vi "Stop Sub-Panel VI.vi"(8 "error in (no error) 2":errorcluster, 11 "reference":refnum<vi>) -> (0 "error IO":errorcluster)   [LabVIEW 2011, in "PXIe-433x Custom Device.lvlib"]
uses:
  PXIe-433x Custom Device.lvlib
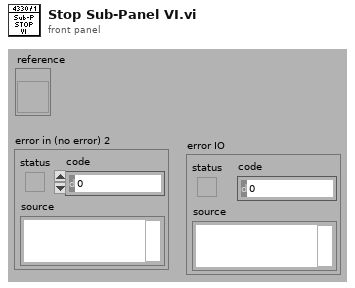
[diagram p1: front panel]
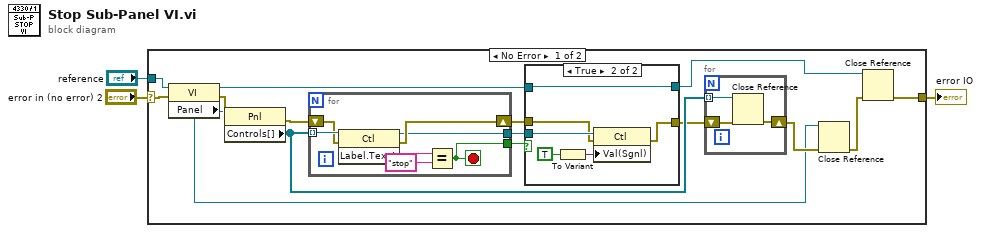
[diagram p0: block diagram]
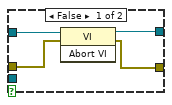
[diagram p2: hidden frame]
diagram:
  n1 = case shown="No Error" "error in (no error) 2" {
    selector: "error in (no error) 2" -> [w6 w39]
    tunnel: [w4 w39] -> w2
    tunnel: "reference" -> [w5 _]
    frame No Error {
      n2 = property class="VI"(reference=w5, error in=w6) -> (reference out=w13:refnum<vi>, error out=w18:errorcluster, "Panel"=w7:refnum<vi>)
      n3 = property class="Pnl"(reference=w7, error in=w18) -> (error out=w17:errorcluster, "Controls[]"=w12:refnum<vi>[])  [unwired: 1 out]
      n4 = for {
        tunnel: w12 -> [w38] mode=indexing
        tunnel: [w35] -> w14
        shift-right: [w33] -> w15
        shift-left: w17 -> [w34]
        tunnel: [w32] -> w16
        stop <- w35 stop-if-true
        n5 = property class="Ctl"(reference=w38, error in=w34) -> (reference out=w32:refnum<vi>, error out=w33:errorcluster, "Label.Text"=w37:string)
        n6 = Equal?(x=w37, y="stop") -> (x = y?=w35:bool)
      }
      n7 = case shown="True" w14 {
        tunnel: w16 -> [_ w31]
        tunnel: w15 -> [w24 w28]
        tunnel: w13 -> [w25 w26]
        tunnel: [w23 w26] -> w11
        tunnel: [w22 w27] -> w10
        frame False {
          n8 = invoke class="VI" method="Abort VI"(reference=w25, error in=w24) -> (reference out=w23:refnum<vi>, error out=w22:errorcluster)  [unwired: 1 in, 1 out]
        }
        frame True {
          n9 = To Variant(anything=TRUE) -> (Variant=w29:variant)
          n10 = property class="Ctl"(reference=w31, error in=w28, "Val(Sgnl)"=w29) -> (error out=w27:errorcluster)  [unwired: 1 out]
        }
      }
      n11 = for {
        tunnel: w12 -> [w21] mode=indexing
        shift-right: [w19] -> w8
        shift-left: w10 -> [w20]
        n12 = Close Reference(reference=w21, error in (no error)=w20) -> (error out=w19:errorcluster)
      }
      n13 = Close Reference(reference=w7, error in (no error)=w8) -> (error out=w9:errorcluster)
      n14 = Close Reference(reference=w11, error in (no error)=w9) -> (error out=w4:errorcluster)
    }
    frame Error {
    }
  }
  "error IO" <- w2
